vi "Serial Host.vi"() -> ()   [LabVIEW 2012]
uses:
  <vilib>/rvi/interface/nirviOpenFPGA/nirviOpenFPGA.xnode
  UART 8N1/sbRIO Example.vi
panel:
  in  "stop":bool
  in  "Data":u8[](array[numeric])
  in  "Write":bool
  out "Elements Remaining":u32
  out "Serial Out":string
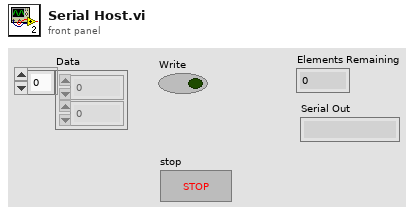
[diagram p1: front panel]
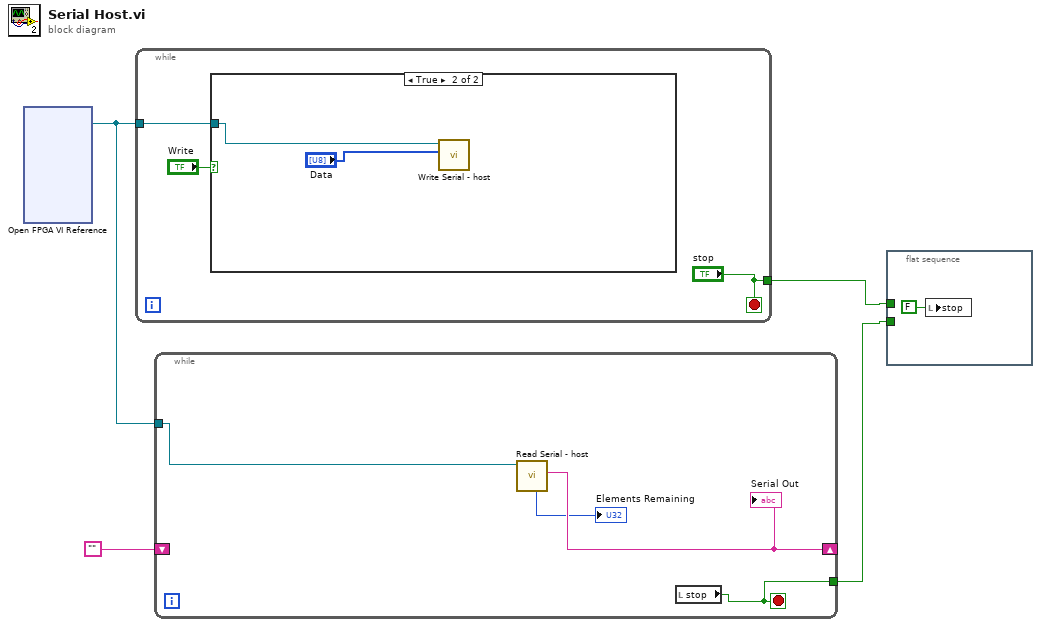
[diagram p0: block diagram]
diagram:
  n1 = xnode "Open FPGA VI Reference"() -> ("FPGA VI Reference Out"=w4:refnum<k20>)  [unwired: 2 in, 1 out]
  n2 = while {
    tunnel: w4 -> [w7]
    tunnel: ["stop"] -> w2
    stop <- "stop" stop-if-true
    n3 = case shown="True" "Write" {
      tunnel: w7 -> [_ w9]
      frame False {
      }
      frame True {
        n4 = call "Write Serial - host.vi"("Data"="Data", "Refnum in"=w9) -> ()  [unwired: 9 in, 1 out]
      }
    }
  }
  n5 = while {
    tunnel: w4 -> [w13]
    shift-right: [w11] -> _
    shift-left: "" -> [_]
    tunnel: [w12] -> w1
    stop <- w12 stop-if-true
    n6 = call "Read Serial - host.vi"("Refnum in"=w13) -> ("String out"=w11:string, "Elements Remaining"=→"Elements Remaining":u32)  [unwired: 8 in, 1 out]
    "Serial Out" <- w11
    n7 = local read "stop"() -> (w12:bool)
  }
  n8 = flat-sequence {
    tunnel: w2 -> [_]
    tunnel: w1 -> [_]
    frame #0 {
      n9 = local write "stop"(FALSE ("stop")) -> ()
    }
  }
